vi "Configure Measurement.vi"   [LabVIEW 2016, in "Keithley 2182A.lvlib"]
uses:
  <instrlib>/Keithley 2182A/Keithley 2182A.lvlib
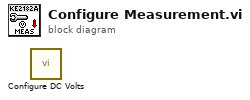
[diagram p0: block diagram]
diagram:
  n1 = call <instrlib>:"Configure DC Volts.vi"() -> ()  [unwired: 10 in, 2 out]
